vi "set_config_cluster.vi"(8 "error in (no error)":errorcluster, 10 "config cluster variant":variant, 11 "ScanHeadMH100729FPGA in":refnum<class "ScanHeadMH100729FPGA.lvclass">) -> (0 "error out":errorcluster, 3 "ScanHeadMH100729FPGA out":refnum<class "ScanHeadMH100729FPGA.lvclass">)   [LabVIEW 2010, in "ScanHeadMH100729FPGA.lvclass"]
uses:
  ScanHeadMH100729FPGA.lvclass
  ScanHeadMH100729FPGA.lvclass/ScanHeadMH100729FPGA.ctl
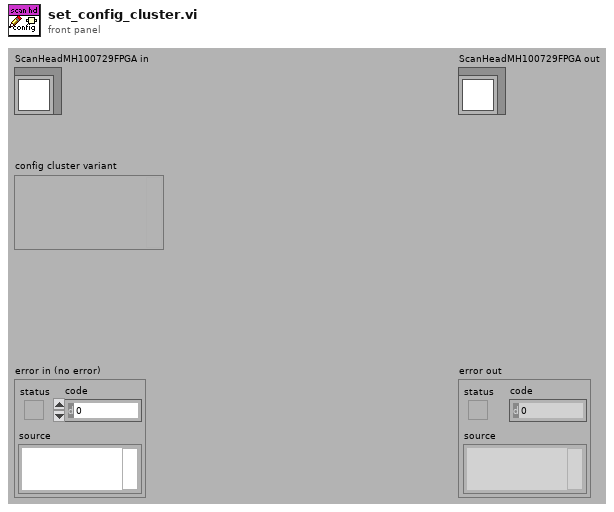
[diagram p1: front panel]
types:
  T1 = typedef "ScanHeadMH100729FPGA.lvclass/config_data_cluster.ctl" = cluster{"LSID":T2, "visibility":cluster{"Zoom":bool, "RotateX":bool, "RotateY":bool, "TranslateX":bool, "TranslateY":bool, "TranslateZ":bool}, "subcomponent specifications":cluster{"intensity modifier":T3, "shutter":T3}, "translation factor":dbl[unit]}
  T2 = typedef "LSID_cluster.ctl" = cluster{"identifier":string, "revision":i32}
  T3 = typedef "plugin_specification.ctl" = cluster{"class path":string, "configuration":string, "label":string, "settings name":string}
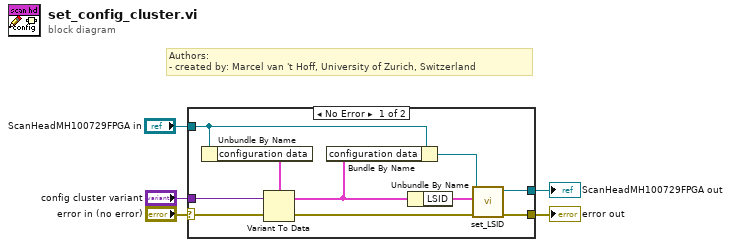
[diagram p0: block diagram]
diagram:
  # "Authors: \n- created by: Marcel van 't Hoff, University of Zurich, Switzerland"
  n1 = case shown="No Error" "error in (no error)" {
    selector: "error in (no error)" -> [w7 w17]
    tunnel: [w8 w17] -> w4
    tunnel: "ScanHeadMH100729FPGA in" -> [w13 w16]
    tunnel: [w9 w16] -> w2
    tunnel: "config cluster variant" -> [w15 _]
    frame No Error {
      n2 = Unbundle By Name(w13) -> ("configuration data"=w14:T1)
      n3 = Variant To Data(error in=w7, Variant=w15, type=w14) -> (error out=w6:errorcluster, data=w12:T1)
      n4 = Bundle By Name(cluster=w13, "configuration data"=w12) -> (w10:refnum<class "ScanHeadMH100729FPGA.lvclass">)
      n5 = Unbundle By Name(w12) -> ("LSID"=w11:T2)
      n6 = call-dynamic "set_LSID.vi"("error in (no error)"=w6, "LSID"=w11, "GenericPlugin in"=w10) -> ("error out"=w8:errorcluster, "GenericPlugin out"=w9:refnum<class "ScanHeadMH100729FPGA.lvclass">)  [unwired: 7 in]
    }
    frame Error {
    }
  }
  "error out" <- w4
  "ScanHeadMH100729FPGA out" <- w2
